vi "niFpga wdp fft output buffer.vi"(4 "enable":bool, 6 "memory switch":bool, 8 "read index":fxp<+,9,9>, 9 "write index":fxp<+,9,9>, 10 "data in 1":T1, 11 "data in 0":T1) -> (2 "data out im":fxp<+/-,8,1>[](array[numeric]), 3 "data out re":fxp<+/-,8,1>[](array[numeric]))   [LabVIEW 2017]
uses:
  <vilib>/rvi/Analysis/measure/FFT/config/niFpgaFFTIOPattern.ctl
  <vilib>/rvi/Emulation/niFpgaSctlEmulationGetInTimedLoop.vi
  <vilib>/Utility/error.llb/Clear Errors.vi
  <vilib>/rvi/DataTransferAndStorage/Container/Common/niFpgaContainerGetUniqueNameForEmu.vi
  <vilib>/rvi/DataTransferAndStorage/Container/Common/niFpgaContainerSetEmuInfo.vi
  <vilib>/rvi/eio/common/nirviEmuReportErrorAndStop.vi
  <vilib>/rvi/DataTransferAndStorage/Container/Common/niFpgaContainerExecOnDevCompGetState.vi
  <vilib>/rvi/Emulation/niFpgaEmulationIsFPGAContextNoSignature.vi
  <vilib>/rvi/Emulation/niFpgaProcessEmulError.vi
  <vilib>/rvi/errors/nirviReportUnexpectedCaseInternalError (U32).vi
  <vilib>/rvi/Memory/Memory_Emulation/niFpgaMemoryEmulationCacheClearOnFirstRun.vi
  <vilib>/rvi/Memory/Memory_Emulation/nirvimemoryEmulationManagerCache_MakeExclusive.vi
  <vilib>/rvi/Memory/Memory_Emulation/niFpgaMemoryEmulationValidateCache.vi
  <vilib>/rvi/Memory/Memory_Emulation/nirvimemoryEmulationManagerCache_InsertValue.vi
  <vilib>/rvi/Memory/Memory_Emulation/nirvimemoryEmulationManagerCache_ReleaseExclusive.vi
  <vilib>/rvi/Memory/Memory_Emulation/nirvimemoryEmulationManagerCache_GetValue.vi
  <vilib>/rvi/Memory/Memory_Emulation/nirvimemoryEmulationManagerCache_SetValue.vi
  <vilib>/rvi/Emulation/niFpgaSctlEmulationResourceMgr.vi
  <vilib>/rvi/LocalResourceManager/LocalResourceManager.xnode
  <vilib>/rvi/DataTransferAndStorage/Container/XNode/niFpgaContainer.xnode
  <vilib>/rvi/Memory/Memory_Emulation/niFpgaMemoryEmulationRefIn.vi
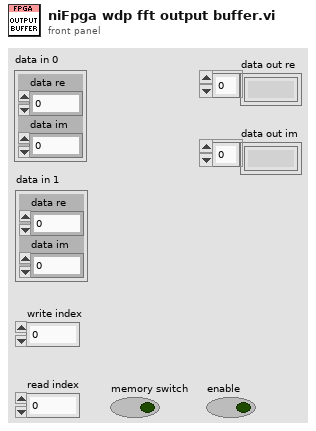
[diagram p1: front panel]
types:
  T1 = cluster{"data re":fxp<+/-,19,1>, "data im":fxp<+/-,19,1>}
  T2 = typedef "niFpgaFFTIOPattern.ctl" = enum16{"CI/CO", "CI/DO", "DI/CO"}
  T3 = cluster{"output data type":fxp<+/-,8,1>, "output data type":fxp<+/-,8,1>}
  T4 = cluster{"dara re":fxp<+/-,8,1>, "dara im":fxp<+/-,8,1>}
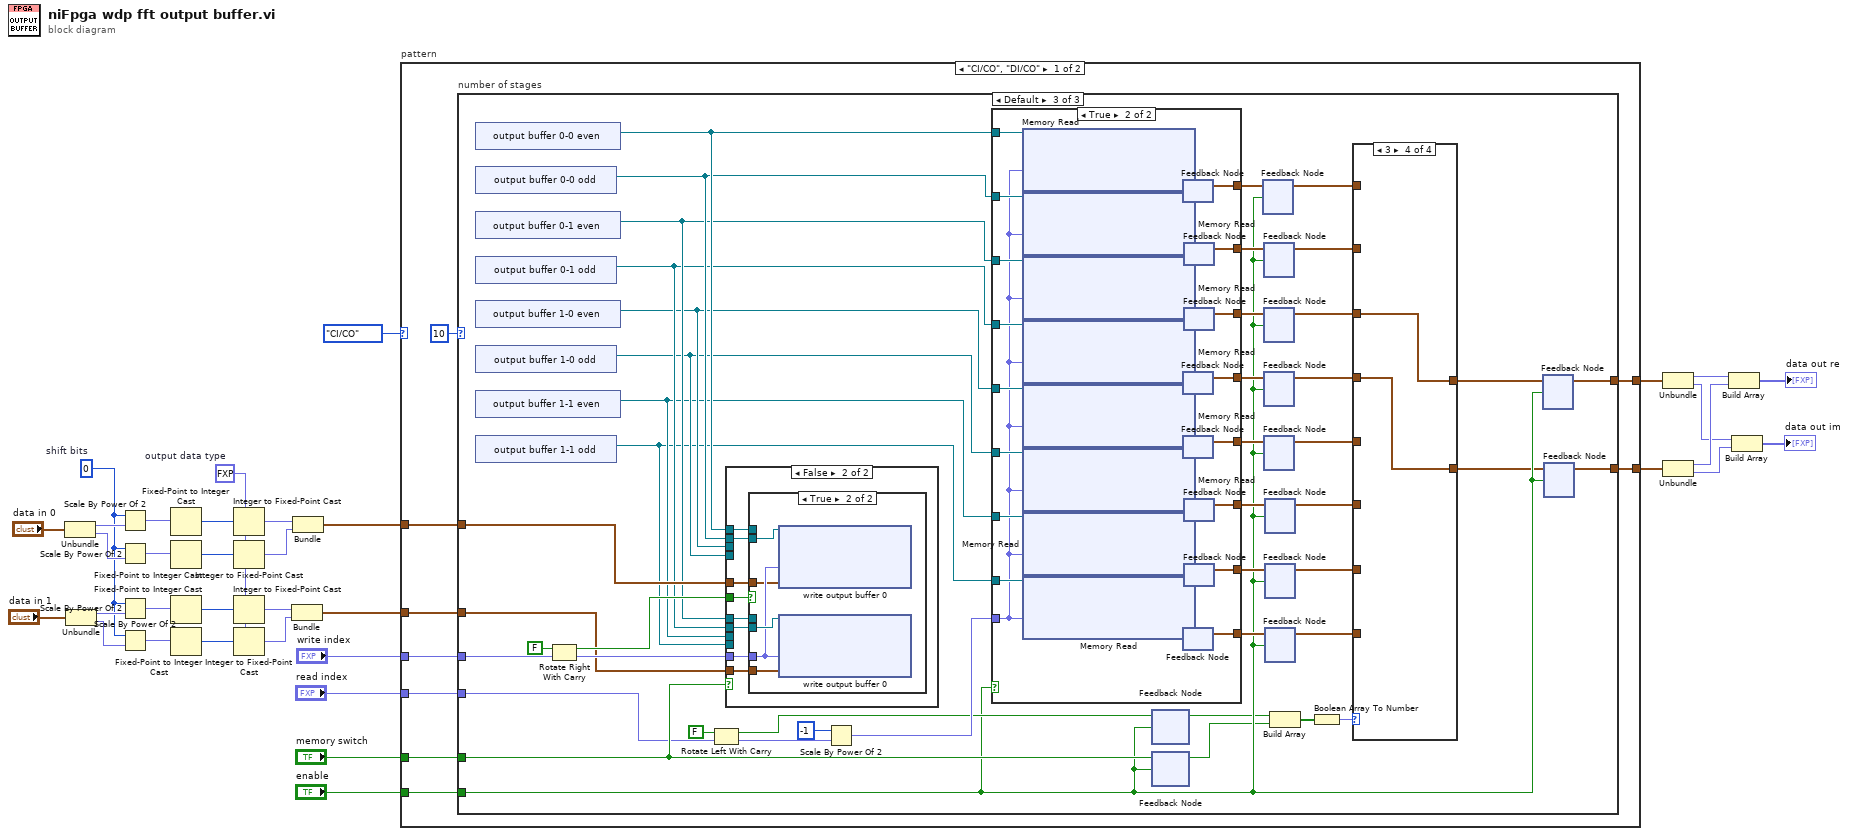
[diagram p0: block diagram]
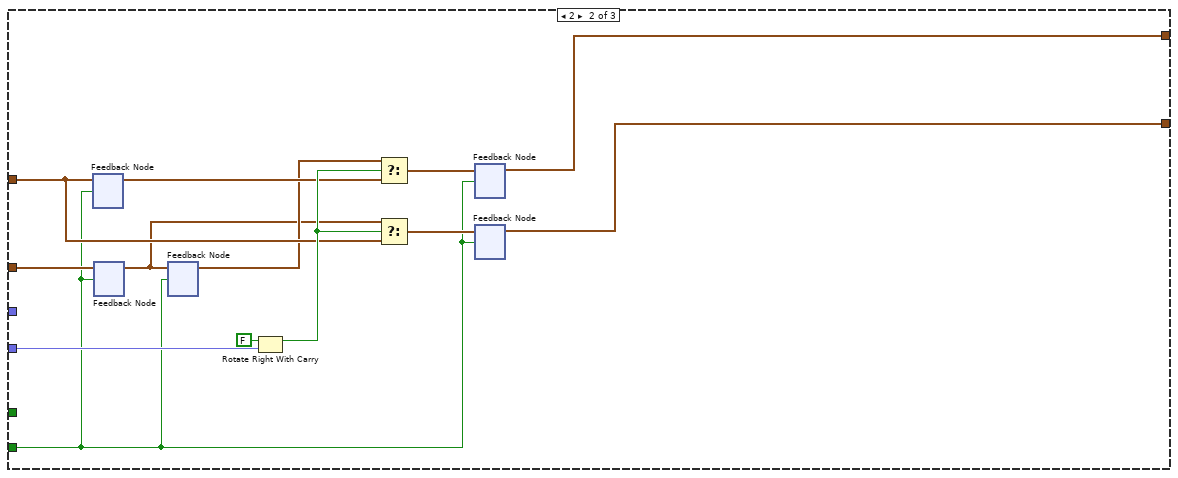
[diagram p3: hidden frame]
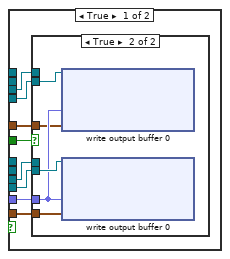
[diagram p8: hidden frame]
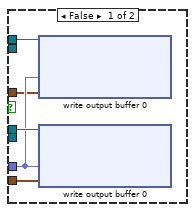
[diagram p9: hidden frame]
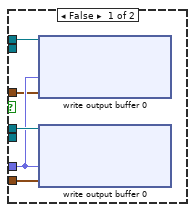
[diagram p10: hidden frame]
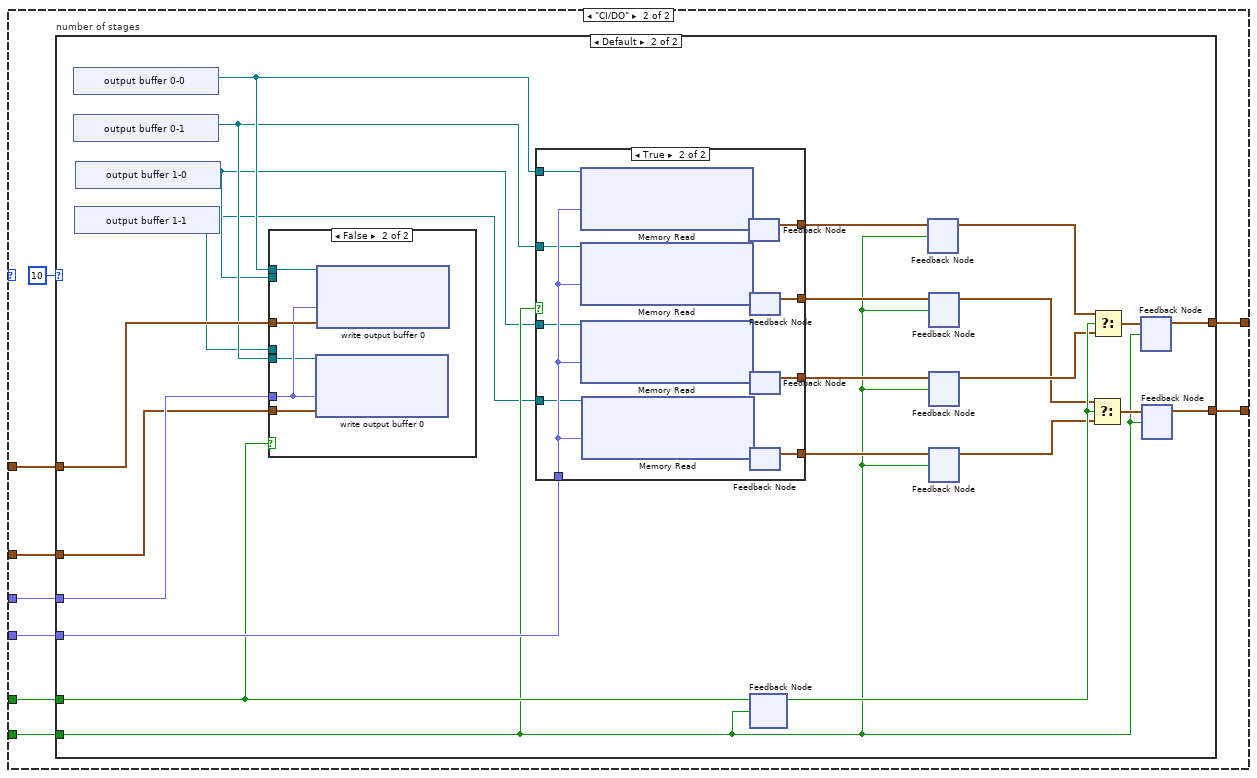
[diagram p11: hidden frame]
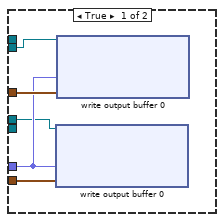
[diagram p14: hidden frame]
diagram:
  w20 = fxp<+/-,8,1> 0.0  # output data type
  w21 = i16 0  # shift bits
  n1 = Unbundle("data in 0") -> ("data re"=w24:fxp<+/-,19,1>, "data im"=w26:fxp<+/-,19,1>)
  n2 = Unbundle("data in 1") -> ("data re"=w29:fxp<+/-,19,1>, "data im"=w30:fxp<+/-,19,1>)
  n3 = Scale By Power Of 2(n=w21, x=w24) -> (x*2^n=w25:fxp<+/-,19,1>)
  n4 = Scale By Power Of 2(n=w21, x=w26) -> (x*2^n=w27:fxp<+/-,19,1>)
  n5 = Scale By Power Of 2(n=w21, x=w29) -> (x*2^n=w28:fxp<+/-,19,1>)
  n6 = Scale By Power Of 2(n=w21, x=w30) -> (x*2^n=w31:fxp<+/-,19,1>)
  n7 = Fixed-Point to Integer Cast(1:w25) -> (0:w19:i32)
  n8 = Fixed-Point to Integer Cast(1:w27) -> (0:w18:i32)
  n9 = Fixed-Point to Integer Cast(1:w28) -> (0:w17:i32)
  n10 = Fixed-Point to Integer Cast(1:w31) -> (0:w16:i32)
  n11 = Integer to Fixed-Point Cast(fixed-point type=w20, integer=w19) -> (fixed-point=w15:fxp<+/-,8,1>)
  n12 = Integer to Fixed-Point Cast(fixed-point type=w20, integer=w18) -> (fixed-point=w14:fxp<+/-,8,1>)
  n13 = Integer to Fixed-Point Cast(fixed-point type=w20, integer=w17) -> (fixed-point=w13:fxp<+/-,8,1>)
  n14 = Integer to Fixed-Point Cast(fixed-point type=w20, integer=w16) -> (fixed-point=w12:fxp<+/-,8,1>)
  n15 = Bundle("output data type"=w13, "output data type"=w12) -> (w10:T3)  [unwired: 1 in]
  n16 = Bundle("output data type"=w15, "output data type"=w14) -> (w11:T3)  [unwired: 1 in]
  n17 = case "pattern" shown="\"CI/CO\", \"DI/CO\"" niFpgaFFTIOPattern."CI/CO" {
    tunnel: "memory switch" -> [w37 w183]
    tunnel: "enable" -> [w36 w182]
    tunnel: "write index" -> [w39 w181]
    tunnel: "read index" -> [w38 w180]
    tunnel: w11 -> [w41 w178]
    tunnel: w10 -> [w42 w177]
    tunnel: [w44 w176] -> w9
    tunnel: [w43 w175] -> w8
    frame "CI/CO", "DI/CO" {
      n18 = case "number of stages" shown="Default" u8 10 {
        tunnel: w41 -> [w46 w54 w99]
        tunnel: w39 -> [_ _ w103]
        tunnel: [w46 w49 w105] -> w44
        tunnel: [w45 w48 w104] -> w43
        tunnel: w38 -> [_ w58 w80]
        tunnel: w37 -> [_ _ w97]
        tunnel: w36 -> [_ w47 w74]
        tunnel: w42 -> [w45 w57 w98]
        frame 0, 1 {
        }
        frame 2 {
          n19 = feedback #1() -> (w55:T3)  [unwired: 1 in]
          n20 = feedback-in #1(w54, w47) -> ()
          n21 = feedback #2() -> (w52:T3)  [unwired: 1 in]
          n22 = feedback-in #2(w57, w47) -> ()
          n23 = feedback #3() -> (w53:T3)  [unwired: 1 in]
          n24 = feedback-in #3(w52, w47) -> ()
          n25 = Rotate Right With Carry(2:w58, 3:FALSE ("carry")) -> (1:w56:bool)  [unwired: 1 out]
          n26 = Select(t=w53, s=w56, f=w55) -> (s? t:f=w51:T3)
          n27 = Select(t=w52, s=w56, f=w54) -> (s? t:f=w50:T3)
          n28 = feedback #4() -> (w49:T3)  [unwired: 1 in]
          n29 = feedback-in #4(w51, w47) -> ()
          n30 = feedback #5() -> (w48:T3)  [unwired: 1 in]
          n31 = feedback-in #5(w50, w47) -> ()
        }
        frame Default {
          n32 = xnode "output buffer 0-0 even"() -> ("Memory Out"=w96:refnum<k21>)
          n33 = xnode "output buffer 0-0 odd"() -> ("Memory Out"=w95:refnum<k21>)
          n34 = xnode "output buffer 0-1 even"() -> ("Memory Out"=w94:refnum<k21>)
          n35 = xnode "output buffer 0-1 odd"() -> ("Memory Out"=w93:refnum<k21>)
          n36 = xnode "output buffer 1-0 even"() -> ("Memory Out"=w92:refnum<k21>)
          n37 = xnode "output buffer 1-0 odd"() -> ("Memory Out"=w91:refnum<k21>)
          n38 = xnode "output buffer 1-1 even"() -> ("Memory Out"=w90:refnum<k21>)
          n39 = xnode "output buffer 1-1 odd"() -> ("Memory Out"=w89:refnum<k21>)
          n40 = Rotate Right With Carry(2:w103, 3:FALSE ("carry")) -> (0:w100:fxp<+,9,9>, 1:w101:bool)
          n41 = Rotate Left With Carry(2:w80, 3:FALSE ("carry")) -> (0:w78:fxp<+,9,9>, 1:w75:bool)
          n42 = case shown="False" w97 {
            tunnel: w96 -> [_ w164]
            tunnel: w92 -> [w146 _]
            tunnel: w95 -> [_ w163]
            tunnel: w93 -> [_ w161]
            tunnel: w91 -> [w145 _]
            tunnel: w94 -> [_ w162]
            tunnel: w90 -> [w144 _]
            tunnel: w89 -> [w143 _]
            tunnel: w101 -> [w142 w160]
            tunnel: w100 -> [w141 w159]
            tunnel: w99 -> [w140 w157]
            tunnel: w98 -> [w139 w158]
            frame True {
              n43 = case shown="True" w142 {
                tunnel: w146 -> [w151 _]
                tunnel: w145 -> [_ w156]
                tunnel: w144 -> [w150 _]
                tunnel: w143 -> [_ w155]
                tunnel: w141 -> [w149 w154]
                tunnel: w140 -> [w148 w153]
                tunnel: w139 -> [w147 w152]
                frame False {
                  n44 = xnode "write output buffer 0"("Address"=w149, "Data"=w148, "Memory In"=w151) -> ()  [unwired: 1 out]
                  n45 = xnode "write output buffer 0"("Address"=w149, "Data"=w147, "Memory In"=w150) -> ()  [unwired: 1 out]
                }
                frame True {
                  n46 = xnode "write output buffer 0"("Address"=w154, "Data"=w153, "Memory In"=w156) -> ()  [unwired: 1 out]
                  n47 = xnode "write output buffer 0"("Address"=w154, "Data"=w152, "Memory In"=w155) -> ()  [unwired: 1 out]
                }
              }
            }
            frame False {
              n48 = case shown="True" w160 {
                tunnel: w164 -> [w169 _]
                tunnel: w163 -> [_ w174]
                tunnel: w162 -> [w168 _]
                tunnel: w161 -> [_ w173]
                tunnel: w159 -> [w167 w172]
                tunnel: w158 -> [w165 w171]
                tunnel: w157 -> [w166 w170]
                frame False {
                  n49 = xnode ("write output buffer 0")("Address"=w167, "Data"=w166, "Memory In"=w169) -> ()  [unwired: 1 out]
                  n50 = xnode ("write output buffer 0")("Address"=w167, "Data"=w165, "Memory In"=w168) -> ()  [unwired: 1 out]
                }
                frame True {
                  n51 = xnode ("write output buffer 0")("Address"=w172, "Data"=w170, "Memory In"=w174) -> ()  [unwired: 1 out]
                  n52 = xnode ("write output buffer 0")("Address"=w172, "Data"=w171, "Memory In"=w173) -> ()  [unwired: 1 out]
                }
              }
            }
          }
          n53 = Scale By Power Of 2(n=i16 -1, x=w78) -> (x*2^n=w76:fxp<+,9,9>)
          n54 = case shown="True" w74 {
            tunnel: w96 -> [_ w130]
            tunnel: w95 -> [_ w129]
            tunnel: w94 -> [_ w128]
            tunnel: w93 -> [_ w127]
            tunnel: w92 -> [_ w126]
            tunnel: w91 -> [_ w125]
            tunnel: w90 -> [_ w124]
            tunnel: w89 -> [_ w123]
            tunnel: [_ w122] -> w88
            tunnel: [_ w121] -> w87
            tunnel: w76 -> [_ w120]
            tunnel: [_ w119] -> w86
            tunnel: [_ w118] -> w85
            tunnel: [_ w117] -> w84
            tunnel: [_ w116] -> w83
            tunnel: [_ w115] -> w82
            tunnel: [_ w114] -> w81
            frame False {
            }
            frame True {
              n55 = xnode ("Memory Read")("Address"=w120, "Memory In"=w130) -> ("Data"=w138:T4)  [unwired: 1 out]
              n56 = xnode ("Memory Read")("Address"=w120, "Memory In"=w129) -> ("Data"=w137:T4)  [unwired: 1 out]
              n57 = xnode ("Memory Read")("Address"=w120, "Memory In"=w128) -> ("Data"=w136:T4)  [unwired: 1 out]
              n58 = xnode ("Memory Read")("Address"=w120, "Memory In"=w127) -> ("Data"=w135:T4)  [unwired: 1 out]
              n59 = xnode ("Memory Read")("Address"=w120, "Memory In"=w126) -> ("Data"=w131:T4)  [unwired: 1 out]
              n60 = xnode ("Memory Read")("Address"=w120, "Memory In"=w125) -> ("Data"=w132:T4)  [unwired: 1 out]
              n61 = xnode ("Memory Read")("Address"=w120, "Memory In"=w124) -> ("Data"=w133:T4)  [unwired: 1 out]
              n62 = xnode ("Memory Read")("Address"=w120, "Memory In"=w123) -> ("Data"=w134:T4)  [unwired: 1 out]
              n63 = feedback #6() -> (w122:T4)  [unwired: 1 in]
              n64 = feedback-in #6(w138) -> ()
              n65 = feedback #7() -> (w118:T4)  [unwired: 1 in]
              n66 = feedback-in #7(w135) -> ()
              n67 = feedback #8() -> (w117:T4)  [unwired: 1 in]
              n68 = feedback-in #8(w131) -> ()
              n69 = feedback #9() -> (w114:T4)  [unwired: 1 in]
              n70 = feedback-in #9(w134) -> ()
              n71 = feedback #10() -> (w121:T4)  [unwired: 1 in]
              n72 = feedback-in #10(w137) -> ()
              n73 = feedback #11() -> (w119:T4)  [unwired: 1 in]
              n74 = feedback-in #11(w136) -> ()
              n75 = feedback #12() -> (w116:T4)  [unwired: 1 in]
              n76 = feedback-in #12(w132) -> ()
              n77 = feedback #13() -> (w115:T4)  [unwired: 1 in]
              n78 = feedback-in #13(w133) -> ()
            }
          }
          n79 = feedback #14() -> (w72:bool)  [unwired: 1 in]
          n80 = feedback-in #14(w75, w74) -> ()
          n81 = feedback #15() -> (w71:bool)  [unwired: 1 in]
          n82 = feedback-in #15(w97, w74) -> ()
          n83 = feedback #16() -> (w73:T4)  [unwired: 1 in]
          n84 = feedback-in #16(w88, w74) -> ()
          n85 = feedback #17() -> (w65:T4)  [unwired: 1 in]
          n86 = feedback-in #17(w87, w74) -> ()
          n87 = feedback #18() -> (w69:T4)  [unwired: 1 in]
          n88 = feedback-in #18(w86, w74) -> ()
          n89 = feedback #19() -> (w64:T4)  [unwired: 1 in]
          n90 = feedback-in #19(w85, w74) -> ()
          n91 = feedback #20() -> (w68:T4)  [unwired: 1 in]
          n92 = feedback-in #20(w84, w74) -> ()
          n93 = feedback #21() -> (w63:T4)  [unwired: 1 in]
          n94 = feedback-in #21(w83, w74) -> ()
          n95 = feedback #22() -> (w67:T4)  [unwired: 1 in]
          n96 = feedback-in #22(w82, w74) -> ()
          n97 = feedback #23() -> (w62:T4)  [unwired: 1 in]
          n98 = feedback-in #23(w81, w74) -> ()
          n99 = Build Array(w72, w71) -> (w70:bool[])
          n100 = Boolean Array To Number(Boolean array=w70) -> (number=w66:fxp<+,2,2>)
          n101 = case shown="3" w66 {
            tunnel: w73 -> [_ _ w111 _]
            tunnel: w69 -> [_ _ _ w113]
            tunnel: w68 -> [w107 _ _ _]
            tunnel: w67 -> [_ w109 _ _]
            tunnel: [w107 w109 w111 w113] -> w61
            tunnel: w65 -> [_ _ w110 _]
            tunnel: w64 -> [_ _ _ w112]
            tunnel: w63 -> [w106 _ _ _]
            tunnel: w62 -> [_ w108 _ _]
            tunnel: [w106 w108 w110 w112] -> w60
            frame 0, Default {
            }
            frame 1 {
            }
            frame 2 {
            }
            frame 3 {
            }
          }
          n102 = feedback #24() -> (w105:T4)  [unwired: 1 in]
          n103 = feedback-in #24(w61, w74) -> ()
          n104 = feedback #25() -> (w104:T4)  [unwired: 1 in]
          n105 = feedback-in #25(w60, w74) -> ()
        }
      }
    }
    frame "CI/DO" {
      n106 = case "number of stages" shown="Default" u8 10 {
        tunnel: w178 -> [w185 w208]
        tunnel: w181 -> [_ w206]
        tunnel: [w185 w204] -> w176
        tunnel: [w184 w202] -> w175
        tunnel: w180 -> [_ w201]
        tunnel: w183 -> [_ w196]
        tunnel: w182 -> [_ w191]
        tunnel: w177 -> [w184 w186]
        frame 0..2 {
        }
        frame Default {
          n107 = xnode "output buffer 0-0"() -> ("Memory Out"=w190:refnum<k21>)
          n108 = xnode "output buffer 0-1"() -> ("Memory Out"=w189:refnum<k21>)
          n109 = xnode "output buffer 1-1"() -> ("Memory Out"=w187:refnum<k21>)
          n110 = xnode "output buffer 1-0"() -> ("Memory Out"=w188:refnum<k21>)
          n111 = case shown="False" w196 {
            tunnel: w208 -> [w226 w231]
            tunnel: w186 -> [w225 w230]
            tunnel: w206 -> [w224 w229]
            tunnel: w190 -> [_ w228]
            tunnel: w189 -> [_ w227]
            tunnel: w188 -> [w223 _]
            tunnel: w187 -> [w222 _]
            frame True {
              n112 = xnode ("write output buffer 0")("Address"=w224, "Data"=w225, "Memory In"=w222) -> ()  [unwired: 1 out]
              n113 = xnode ("write output buffer 0")("Address"=w224, "Data"=w226, "Memory In"=w223) -> ()  [unwired: 1 out]
            }
            frame False {
              n114 = xnode ("write output buffer 0")("Address"=w229, "Data"=w230, "Memory In"=w227) -> ()  [unwired: 1 out]
              n115 = xnode ("write output buffer 0")("Address"=w229, "Data"=w231, "Memory In"=w228) -> ()  [unwired: 1 out]
            }
          }
          n116 = case shown="True" w191 {
            tunnel: w201 -> [_ w221]
            tunnel: [_ w216] -> w200
            tunnel: [_ w215] -> w199
            tunnel: [_ w214] -> w198
            tunnel: [_ w213] -> w197
            tunnel: w190 -> [_ w212]
            tunnel: w189 -> [_ w211]
            tunnel: w188 -> [_ w210]
            tunnel: w187 -> [_ w209]
            frame False {
            }
            frame True {
              n117 = xnode ("Memory Read")("Address"=w221, "Memory In"=w212) -> ("Data"=w220:T4)  [unwired: 1 out]
              n118 = xnode ("Memory Read")("Address"=w221, "Memory In"=w211) -> ("Data"=w219:T4)  [unwired: 1 out]
              n119 = xnode ("Memory Read")("Address"=w221, "Memory In"=w210) -> ("Data"=w218:T4)  [unwired: 1 out]
              n120 = xnode ("Memory Read")("Address"=w221, "Memory In"=w209) -> ("Data"=w217:T4)  [unwired: 1 out]
              n121 = feedback #26() -> (w216:T4)  [unwired: 1 in]
              n122 = feedback-in #26(w220) -> ()
              n123 = feedback #27() -> (w215:T4)  [unwired: 1 in]
              n124 = feedback-in #27(w219) -> ()
              n125 = feedback #28() -> (w214:T4)  [unwired: 1 in]
              n126 = feedback-in #28(w218) -> ()
              n127 = feedback #29() -> (w213:T4)  [unwired: 1 in]
              n128 = feedback-in #29(w217) -> ()
            }
          }
          n129 = feedback #30() -> (w207:bool)  [unwired: 1 in]
          n130 = feedback-in #30(w196, w191) -> ()
          n131 = feedback #31() -> (w195:T4)  [unwired: 1 in]
          n132 = feedback-in #31(w200, w191) -> ()
          n133 = feedback #32() -> (w193:T4)  [unwired: 1 in]
          n134 = feedback-in #32(w199, w191) -> ()
          n135 = feedback #33() -> (w194:T4)  [unwired: 1 in]
          n136 = feedback-in #33(w198, w191) -> ()
          n137 = feedback #34() -> (w192:T4)  [unwired: 1 in]
          n138 = feedback-in #34(w197, w191) -> ()
          n139 = Select(t=w193, s=w207, f=w192) -> (s? t:f=w203:T4)
          n140 = Select(t=w195, s=w207, f=w194) -> (s? t:f=w205:T4)
          n141 = feedback #35() -> (w204:T4)  [unwired: 1 in]
          n142 = feedback-in #35(w205, w191) -> ()
          n143 = feedback #36() -> (w202:T4)  [unwired: 1 in]
          n144 = feedback-in #36(w203, w191) -> ()
        }
      }
    }
  }
  n145 = Unbundle(w9) -> ("dara re"=w7:fxp<+/-,8,1>, "dara im"=w5:fxp<+/-,8,1>)
  n146 = Unbundle(w8) -> ("dara re"=w6:fxp<+/-,8,1>, "dara im"=w4:fxp<+/-,8,1>)
  n147 = Build Array(w7, w6) -> (→"data out re":fxp<+/-,8,1>[])
  n148 = Build Array(w5, w4) -> (→"data out im":fxp<+/-,8,1>[])
